vi "Set Collection - Word Counting.vi"() -> ()   [LabVIEW 2023]
doc: "This VI demonstrates basic use of the set data type. Sets are used to create a collection of elements. Every element is unique in the set. It is fast to check whether a set contains a given element and easy to iterate over all the elements in sorted order.\n\nThis example uses sets to identify the unique words in two blocks of text and show the overlap of those sets."
uses:
  214e2411-e885-4139-af83-e02a11493df7.vi
  cb11257e-e248-458f-bcf0-1ca918c3c020.vi
  e54fb21d-341e-46d8-a21e-cf9099815c20.vi
  64db6fbb-dfd0-483e-b932-8baaad96f575.vi
panel:
  out "set intersection\n(elements appearing in both sets)":set{string}(c389)
  out "set symmetric difference\n(elements appearing in only one set)":set{string}(c389)
  out "set difference\n(first set minus second set)":set{string}(c389)
  out "second set":set{string}(c389)
  out "first set":set{string}(c389)
  out "set union\n(first set plus second set)":set{string}(c389)
  in  "Second Text":string="c j k l x"
  in  "First Text":string="a b c x y z"
  # "Overview: This VI demonstrates basic use of the set data type. Sets are used to create a collection of elements. Every element is unique in the set. It is fast to check whether a set contains a given element and easy to iterate over all the elements in sorted order.\n\nThis example uses sets to identify the unique words in two blocks of text and show the overlap of those sets.\n\nInstructions:\n1. (optional) Change the sample text in the two string controls.\n2. Run the VI.  \n3. Observe the output: the various set indicators show the unique words found in each block of text, the words that are common to both sets, and the words that are unique to one or the other (the symmetric difference). \n4. Open the block diagram and review further commentary there."
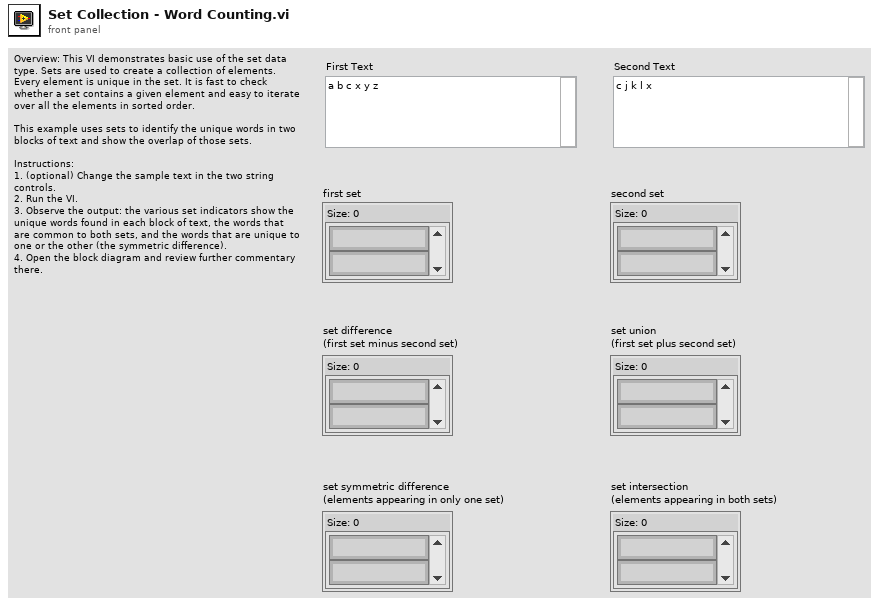
[diagram p1: front panel]
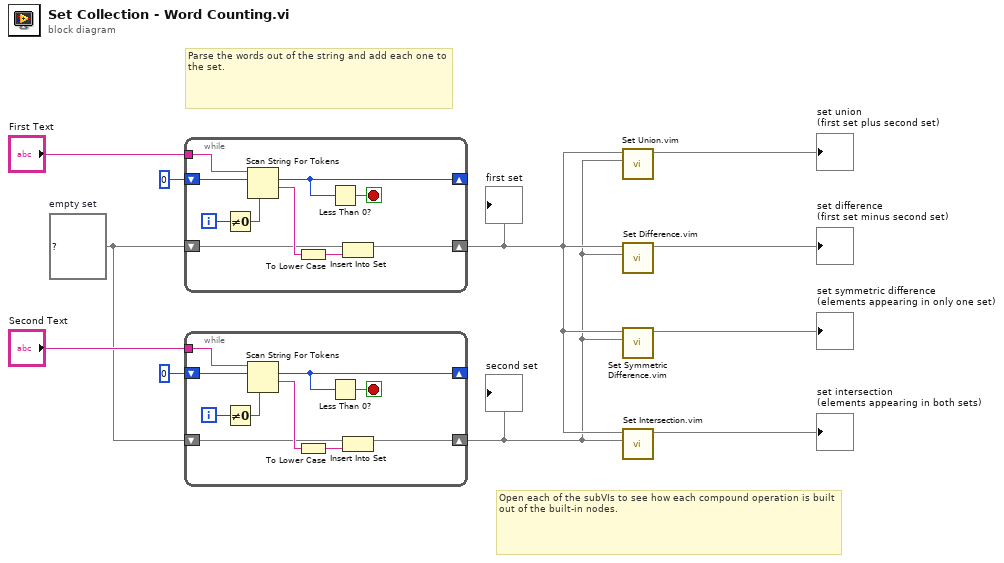
[diagram p0: block diagram]
diagram:
  w7 = set{string} {}  # empty set
  # "Open each of the subVIs to see how each compound operation is built out of the built-in nodes."
  # "Parse the words out of the string and add each one to the set."
  n1 = while {
    tunnel: "First Text" -> [w20]
    shift-left: 0 ("offset past token") -> [w21]
    shift-right: [w15] -> _
    shift-right: [w13] -> w2
    shift-left: w7 -> [w12]
    i -> [w18]
    stop <- w19 stop-if-true
    # "Parse each word."
    n2 = Not Equal To 0?(x=w18) -> (x != 0?=w17:bool)
    n3 = Scan String For Tokens(4:w17, 8:w21, 9:w20) -> (1:w16:string, 2:w15:i32)  [unwired: 3 in, 2 out]
    n4 = To Lower Case(string=w16) -> (all lower case string=w14:string)
    n5 = Less Than 0?(x=w15) -> (x < 0?=w19:bool)
    n6 = Insert Into Set(10:w14, 11:w12) -> (3:w13:set{string})  [unwired: 1 out]
  }
  "first set" <- w2
  n7 = while {
    tunnel: "Second Text" -> [w30]
    shift-left: 0 ("offset past token") -> [w31]
    shift-right: [w25] -> _
    shift-right: [w23] -> w1
    shift-left: w7 -> [w22]
    i -> [w28]
    stop <- w29 stop-if-true
    # "Parse each word."
    n8 = Not Equal To 0?(x=w28) -> (x != 0?=w27:bool)
    n9 = Scan String For Tokens(4:w27, 8:w31, 9:w30) -> (1:w26:string, 2:w25:i32)  [unwired: 3 in, 2 out]
    n10 = To Lower Case(string=w26) -> (all lower case string=w24:string)
    n11 = Less Than 0?(x=w25) -> (x < 0?=w29:bool)
    n12 = Insert Into Set(10:w24, 11:w22) -> (3:w23:set{string})  [unwired: 1 out]
  }
  "second set" <- w1
  n13 = call "Set Union.vim"("set 2"=w1, "set 1"=w2) -> ("union"=→"set union\n(first set plus second set)":set{string})  [unwired: 9 in]
  n14 = call "Set Difference.vim"("set 2"=w1, "set 1"=w2) -> ("difference"=→"set difference\n(first set minus second set)":set{string})  [unwired: 9 in]
  n15 = call "Set Symmetric Difference.vim"("set 2"=w1, "set 1"=w2) -> ("symmetric difference"=→"set symmetric difference\n(elements appearing in only one set)":set{string})  [unwired: 9 in]
  n16 = call "Set Intersection.vim"("set 2"=w1, "set 1"=w2) -> ("intersection"=→"set intersection\n(elements appearing in both sets)":set{string})  [unwired: 9 in]
